vi "Multirecord Acquisition (FPGA) - custom trigger.vi"() -> ()   [LabVIEW 2021]
doc: "Use this VI as a template for the reconfigurable oscilloscope acquisition design. The block diagram is divided into three main loops.\n\nRegister Bus: This loop initializes the registers that are needed to support the configuration of the device. The FIFO bus, on the left, allows all the other design libraries to communicate with one another. This loop is very important to support the proper behavior of the instrument design library components.\n\nAcquisition: Acquires data from the I/O channels and writes the data into the record memory using the <B>Write</B> VI of the Multirecord Acquisition instrument design library. This VI also evaluates the various acquisition triggers and decides whether to acquire each data value in record memory. The host level VI (Fetch Record.vi) can read acquired records from the DRAM. The data is stored in 2 DRAM banks, each with 768 MB of storage.\n\nFetch: The recorded data is retrieved when the <B>Fetch Single Record</B> VI is run from the host VI. The <B>Write to Fetch DMA FIFO</B> VI writes data to the acq.fetch fifo 0 to transmit record data form the FPGA to the record fetch VIs on the host. This DMA FIFO must have a predefined name based on the instance parameter. By default, it is 0 (since the associated terminal on the <B>Create Resources DRAM Write Read</B> VI is unwired), so the connected FIFO is named acq.fetch fifo 0."
uses:
  Trigger/SubVIs/Types/Trigger Type.ctl
  <instrlib>/_niInstr/Data Trigger/v1/Shared/Public/Level Configuration FXP(+-,18,1).ctl
  <instrlib>/_niInstr/Data Trigger/v1/Shared/Public/Level Configuration Trigger When.ctl
  <instrlib>/_niInstr/Data Trigger/v1/Shared/Public/Edge Configuration FXP(+-,18,1).ctl
  <instrlib>/_niInstr/Data Trigger/v1/Shared/Public/Edge Configuration Trigger Slope.ctl
  FPGA Interface Typedefinitions/Trigger Combination Type.ctl
  Custom Trigger Settings.ctl
  <vilib>/Platform/TimedLoop/XDataNode/timing_clust.ctl
  <vilib>/Platform/TimedLoop/XDataNode/nitl_modes.ctl
  <vilib>/Platform/TimedLoop/XDataNode/wakeup.ctl
  <instrlib>/_niInstr/FIFO Register Bus/v1/FPGA/niInstr FIFO Register Bus v1 FPGA.lvclass
  C:/Program Files (x86)/National Instruments/LabVIEW 2021/instr.lib/_niInstr/Instruction Framework/v1/FPGA/Interfaces/Instruction Producer/Instruction Producer.lvclass
  <vilib>/rvi/Emulation/niFpgaSctlEmulationGetInTimedLoop.vi
  <vilib>/rvi/Emulation/niFpgaEmulationReportErrorSimple.vi
  <vilib>/rvi/Emulation/niFpgaGetClockAttributes.vi
  <vilib>/rvi/Emulation/niFpgaCriticalErrorInLSC.vi
  <vilib>/rvi/eio/common/nirviEmuTemplateMethod_errors.vi
  <instrlib>/HSAI-RIO/Config/Group A/v1/FPGA/Digital Correction/Validate 8 Channel Data.vi
  <instrlib>/HSAI-RIO/Config/Group A/v1/FPGA/Digital Correction/Digital Correction (8 Ch).vi
  <instrlib>/HSAI-RIO/Config/Group A/v1/FPGA/Digital Correction/FIR Filter (8 Ch).vi
  DSP/SubVIs/Integer decimationx8ch.vi
  Data Type Conversion/SubVIs/Remove Overflow FXP(+-,18,1)x8ch.vi
  Data Type Conversion/SubVIs/Data Type Conversion FXP(+-,18,1) to I16x8ch.vi
  <vilib>/Platform/TimedLoop/XDataNode/XDataNode.xnode
  <instrlib>/_niInstr/Instruction Framework/v1/FPGA/Interfaces/Address Space Collection/Address Space Collection.lvclass
  <instrlib>/_niInstr/Multirecord Acquisition/Common/v1/FPGA/niInstr Multirecord Acquisition Common v1 FPGA.lvclass
  <vilib>/eio/EIONode/EIONode.xnode
  <instrlib>/_niInstr/Instruction Framework/v1/FPGA/Top Level Bus/Register Configuration/Register Configuration.lvclass
  <vilib>/Platform/TimedLoop/XDataNode/XDNodeRunTimeDep.lvlib
  <vilib>/rvi/LocalResourceManager/LocalResourceManager.xnode
  <vilib>/rvi/eio/common/nirviEmuReportErrorAndStop.vi
  <vilib>/rvi/DataTransferAndStorage/Container/Common/niFpgaContainerGetUniqueNameForEmu.vi
  <vilib>/rvi/DataTransferAndStorage/Container/Common/niFpgaContainerSetEmuInfo.vi
  <instrlib>/_niInstr/Basic Elements/v1/FPGA/niInstr Basic Elements v1 FPGA.lvlib
  <instrlib>/_niInstr/Multirecord Acquisition/Common/v1/FPGA/Private/Create Fetch DMA FIFO Resources U8x32.vi
  <instrlib>/HSAI-RIO/Config/Group A/v1/FPGA/Digital Correction/Digital Correction.lvclass
  <instrlib>/HSAI-RIO/Config/Group A/v1/FPGA/Config Registers/Config Registers.lvclass
  <instrlib>/_niInstr/Multirecord Acquisition/Common/v1/FPGA/Private/Create Resources BRAM U384.vi
  <instrlib>/_niInstr/Multirecord Acquisition/Common/v1/FPGA/Private/Create Resources DRAM U384.vi
  <instrlib>/_niInstr/Multirecord Acquisition/Common/v1/FPGA/Private/Create Resources BRAM U768.vi
  Emulation/SubVIs/2 Element Generate Sine Cos Data FXP(+,-,14,1).vi
  C:/Program Files (x86)/National Instruments/LabVIEW 2021/instr.lib/_niInstr/FIFO Register Bus/v1/FPGA/niInstr FIFO Register Bus v1 FPGA.lvclass
  <instrlib>/_niInstr/Data Trigger/v1/Shared/niInstr Data Trigger v1 Shared.lvlib
  FPGA Interface Typedefinitions/FPGA Interface Typedefinitions.lvlib
panel:
  in  "Trigger Settings 7":T1
  in  "Trigger Settings 6":T1
  in  "Trigger Settings 5":T1
  in  "Trigger Settings 4":T1
  in  "Trigger Settings 3":T1
  in  "Trigger Settings 2":T1
  in  "Trigger Settings 1":T1
  in  "Trigger Settings 0":T1
  in  "trigger.rearm delay":u16=2
  in  "start trigger":bool=TRUE
  in  "trigger.type B":T2
  in  "reset":bool
  in  "trigger.combination type":T3
  in  "trigger.edge B":T4
  in  "trigger.level B":T6
  in  "trigger.edge A":T4
  in  "trigger.level A":T6
  in  "trigger.type A":T2
  in  "trigger.channel A":u8
  in  "trigger.channel B":u8
  out "fifo reg bus data 0":u64
  out "fifo reg bus status 0":u32
  in  "fifo reg bus ctrl 0":u32
  out "overflow":bool
  in  "dsp.decimation factor":u16
  out "overload":bool
  in  "channel.enable mask":u16=65535 format="%.0b"
  in  "channel.number of channels":u8=8
  # "Register Bus Controls"
  # "FPGA"
  # "Acquisition Loop Controls"
  # "DSP"
  # "Trigger"
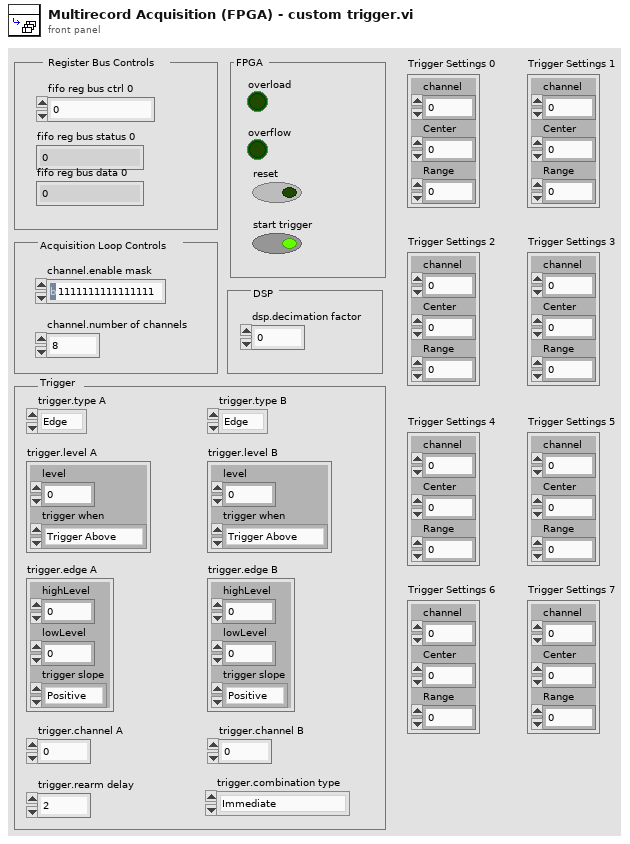
[diagram p1: front panel]
types:
  T1 = typedef "Custom Trigger Settings.ctl" = cluster{"channel":u8, "Center":fxp<+/-,24,1>, "Range":fxp<+,24,1>}
  T2 = typedef "Trigger Type.ctl" = enum16{"Edge", "Level", "Custom"}
  T3 = typedef "FPGA Interface Typedefinitions.lvlib/Trigger Combination Type.ctl" = enum16{"Immediate", "A", "B", "OR", "AND", "A THEN B", "B THEN A", "High Resolution"}
  T4 = typedef "niInstr Data Trigger v1 Shared.lvlib/Edge Configuration FXP(+-,18,1).ctl" = cluster{"highLevel":fxp<+/-,18,1>, "lowLevel":fxp<+/-,18,1>, "trigger slope":T5}
  T5 = typedef "niInstr Data Trigger v1 Shared.lvlib/Edge Configuration Trigger Slope.ctl" = enum8{"Positive", "Negative"}
  T6 = typedef "niInstr Data Trigger v1 Shared.lvlib/Level Configuration FXP(+-,18,1).ctl" = cluster{"level":fxp<+/-,18,1>, "trigger when":T7}
  T7 = typedef "niInstr Data Trigger v1 Shared.lvlib/Level Configuration Trigger When.ctl" = enum8{"Trigger Above", "Trigger Below"}
  T8 = cluster{"memory 1":refnum<k21>, "memory 2":refnum<k21>}
  T9 = typedef "XDNodeRunTimeDep.lvlib/timing_clust.ctl" = cluster{"Expected End [f-1]":u64, "Actual End [f-1]":u64, "Finished Late? [f-1]":bool, "Expected End [i-1]":u64, "Actual End [i-1]":u64, "Finished Late? [i-1]":bool, "Expected Start [i]":u64, "Actual Start [i]":u64, "Expected Start [f]":u64, "Actual Start [f]":u64, "Source Name":string, "Structure Name":string, "Period":i64, "Deadline":i64, "Offset":i64, "Start":i64, "Priority":i32, "Timeout":i32, "Mode":T10, "Wakeup Reason":T11, "Error":errorcluster, "Source Type":string, "Secondary Source Type":string, "Global End Time":u64, "Global Start Time":u64, "Frame Duration":u64, "Iteration Duration":u64, "Assigned CPU":i32, "I/O Scan Engine Mode":u32}
  T10 = typedef "XDNodeRunTimeDep.lvlib/nitl_modes.ctl" = enum32{"No Change", "Process missed periods, maintain original phase", "Discard missed periods, maintain original phase", "Process missed periods, ignore original phase", "Discard missed periods, ignore original phase"}
  T11 = typedef "XDNodeRunTimeDep.lvlib/wakeup.ctl" = enum32{"Normal", "Aborted", "Asynchronous wakeup", "Timing source error", "Timed loop error", "Timeout"}
  T12 = cluster{"Channel 0":fxp<+/-,14,1>[], "Channel 1":fxp<+/-,14,1>[], "Channel 2":fxp<+/-,14,1>[], "Channel 3":fxp<+/-,14,1>[], "Channel 4":fxp<+/-,14,1>[], "Channel 5":fxp<+/-,14,1>[], "Channel 6":fxp<+/-,14,1>[], "Channel 7":fxp<+/-,14,1>[]}
  T13 = cluster{"Channel 0":fxp<+/-,18,1>[], "Channel 1":fxp<+/-,18,1>[], "Channel 2":fxp<+/-,18,1>[], "Channel 3":fxp<+/-,18,1>[], "Channel 4":fxp<+/-,18,1>[], "Channel 5":fxp<+/-,18,1>[], "Channel 6":fxp<+/-,18,1>[], "Channel 7":fxp<+/-,18,1>[]}
  T14 = cluster{"channel 0":fxp<+/-,18,1>[], "channel 1":fxp<+/-,18,1>[], "channel 2":fxp<+/-,18,1>[], "channel 3":fxp<+/-,18,1>[], "channel 4":fxp<+/-,18,1>[], "channel 5":fxp<+/-,18,1>[], "channel 6":fxp<+/-,18,1>[], "channel 7":fxp<+/-,18,1>[]}
  T15 = cluster{"channel 0":i16[], "channel 1":i16[], "channel 2":i16[], "channel 3":i16[], "channel 4":i16[], "channel 5":i16[], "channel 6":i16[], "channel 7":i16[]}
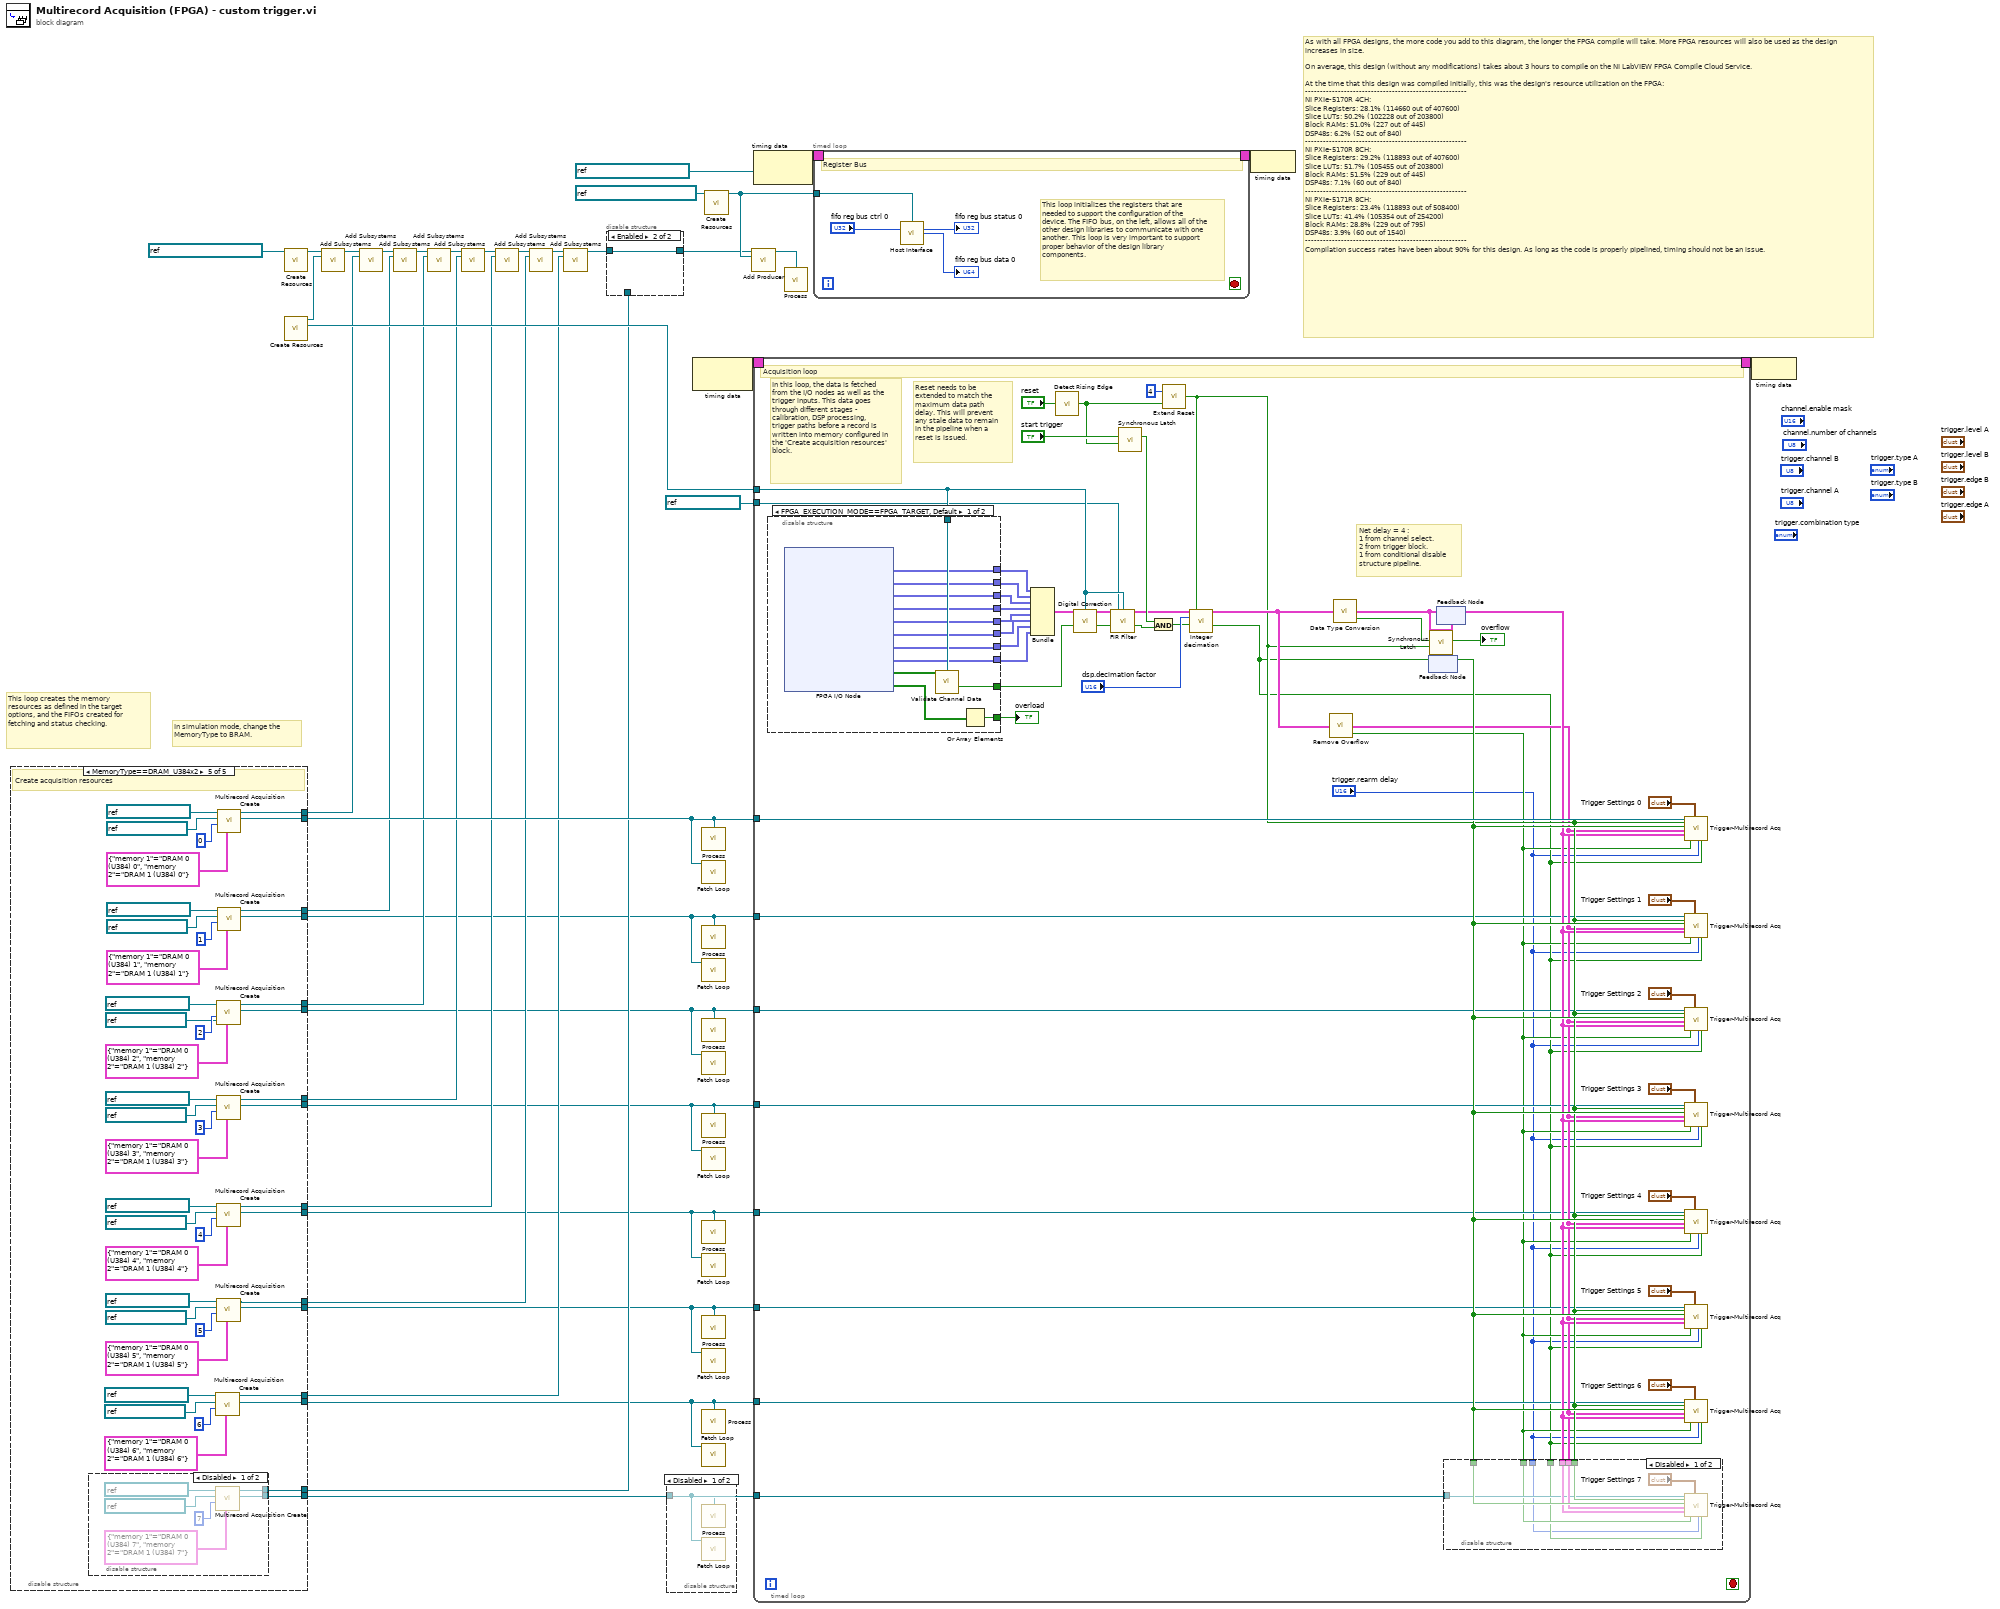
[diagram p0: block diagram]
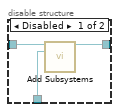
[diagram p2: hidden frame]
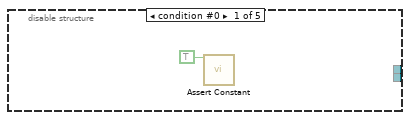
[diagram p4: hidden frame]
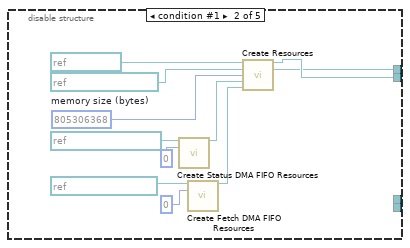
[diagram p5: hidden frame]
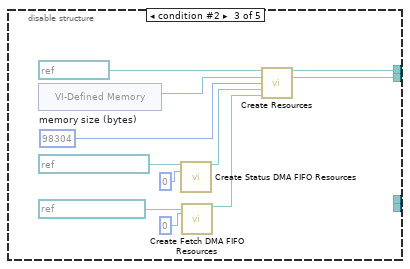
[diagram p6: hidden frame]
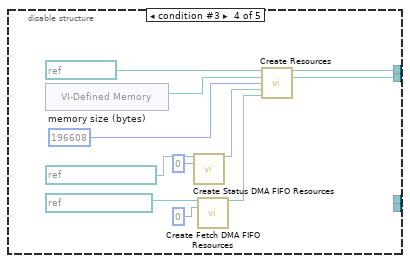
[diagram p7: hidden frame]
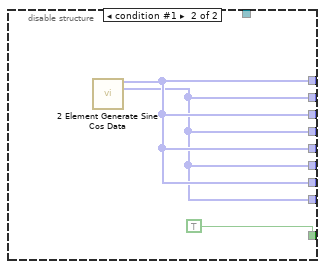
[diagram p10: hidden frame]
diagram:
  # "In simulation mode, change the MemoryType to BRAM."
  # "This loop creates the memory resources as defined in the target options, and the FIFOs created for fetching and status checking."
  # "As with all FPGA designs, the more code you add to this diagram, the longer the FPGA compile will take. More FPGA resources will also be used as the design increases in size.\n\nOn average, this design (without any modifications) takes about 3 hours to compile on the NI LabVIEW FPGA Compile Cloud Service. \n\nAt the time that this design was compiled initially, this was the design's resource utilization on the FPGA:\n------------------------------------------------------\nNI PXIe-5170R 4CH:\nSlice Registers: 28.1% (114660 out of 407600)\nSlice LUTs: 50.2% (102228 out of 203800)\nBlock RAMs: 51.0% (227 out of 445)\nDSP48s: 6.2% (52 out of 840)\n------------------------------------------------------\nNI PXIe-5170R 8CH:\nSlice Registers: 29.2% (118893 out of 407600)\nSlice LUTs: 51.7% (105455 out of 203800)\nBlock RAMs: 51.5% (229 out of 445)\nDSP48s: 7.1% (60 out of 840)\n------------------------------------------------------\nNI PXIe-5171R 8CH:\nSlice Registers: 23.4% (118893 out of 508400)\nSlice LUTs: 41.4% (105354 out of 254200)\nBlock RAMs: 28.8% (229 out of 795)\nDSP48s: 3.9% (60 out of 1540)\n------------------------------------------------------\nCompilation success rates have been about 90% for this design. As long as the code is properly pipelined, timing should not be an issue."
  n1 = disable-structure shown="MemoryType==DRAM_U384x2" {
    disable-tunnel: [_ w48 w59 w70 w116] -> w24
    disable-tunnel: [_ w45 w55 w66 w114] -> w23
    disable-tunnel: [_ _ _ _ w98] -> w22
    disable-tunnel: [_ _ _ _ w97] -> w2
    disable-tunnel: [_ _ _ _ w96] -> w16
    disable-tunnel: [_ _ _ _ w95] -> w3
    disable-tunnel: [_ _ _ _ w94] -> w14
    disable-tunnel: [_ _ _ _ w93] -> w4
    disable-tunnel: [_ _ _ _ w92] -> w13
    disable-tunnel: [_ _ _ _ w91] -> w5
    disable-tunnel: [_ _ _ _ w90] -> w12
    disable-tunnel: [_ _ _ _ w89] -> w6
    disable-tunnel: [_ _ _ _ w88] -> w11
    disable-tunnel: [_ _ _ _ w87] -> w7
    disable-tunnel: [_ _ _ _ w86] -> w9
    disable-tunnel: [_ _ _ _ w85] -> w8
    frame condition #0 {
      n2 = call <instrlib>:"Assert Constant.vi"("constant terminal"=TRUE) -> ()  [unwired: 15 in]
    }
    frame condition #1 {
      w49 = u64 805306368  # memory size (bytes)
      n3 = call <instrlib>:"Create Status DMA FIFO Resources.vi"("status dma fifo in"=refnum<k21> "acq.status fifo 0" ("status dma fifo"), "fifo instance"=u8 0) -> ("status dma fifo out"=w40:refnum<class "niInstr Status FIFO v1 FPGA.lvclass">)  [unwired: 13 in]
      n4 = call-poly <instrlib>:"Create Fetch DMA FIFO Resources.vi"("fetch dma fifo in"=refnum<k21> "acq.fetch fifo 0", "fifo instance"=u8 0) -> ("fetch dma fifo out"=w46:refnum<class "niInstr Fetch FIFO v1 FPGA.lvclass">)  [unwired: 13 in]
      n5 = call-poly <instrlib>:"Create Resources.vi"("memory clock"=refnum<k21> "160MHz" ("process clock"), "memory"=refnum<k21> "DRAM 0 (U384)" ("dram"), "memory size (bytes)"=w49, "status dma fifo resources"=w40, "fetch dma fifo resources"=w46) -> ("acquisition resources"=w48:refnum<class "niInstr Multirecord Acquisition Common v1 FPGA.lvclass">, "acquisition subsystem"=w45:refnum<class "Address Space Collection.lvclass">)  [unwired: 9 in]
    }
    frame condition #2 {
      w60 = u64 98304  # memory size (bytes)
      n6 = xnode "VI-Defined Memory"() -> ("Memory Out"=w61:refnum<k21>)
      n7 = call <instrlib>:"Create Status DMA FIFO Resources.vi"("status dma fifo in"=refnum<k21> "acq.status fifo 0" ("status dma fifo"), "fifo instance"=u8 0) -> ("status dma fifo out"=w52:refnum<class "niInstr Status FIFO v1 FPGA.lvclass">)  [unwired: 13 in]
      n8 = call-poly <instrlib>:"Create Fetch DMA FIFO Resources.vi"("fetch dma fifo in"=refnum<k21> "acq.fetch fifo 0", "fifo instance"=u8 0) -> ("fetch dma fifo out"=w56:refnum<class "niInstr Fetch FIFO v1 FPGA.lvclass">)  [unwired: 13 in]
      n9 = call-poly <instrlib>:"Create Resources.vi"("memory clock"=refnum<k21> "160MHz" ("process clock"), "memory"=w61, "memory size (bytes)"=w60, "status dma fifo resources"=w52, "fetch dma fifo resources"=w56) -> ("acquisition resources"=w59:refnum<class "niInstr Multirecord Acquisition Common v1 FPGA.lvclass">, "acquisition subsystem"=w55:refnum<class "Address Space Collection.lvclass">)  [unwired: 9 in]
    }
    frame condition #3 {
      w71 = u64 196608  # memory size (bytes)
      n10 = xnode "VI-Defined Memory"() -> ("Memory Out"=w72:refnum<k21>)
      n11 = call <instrlib>:"Create Status DMA FIFO Resources.vi"("status dma fifo in"=refnum<k21> "acq.status fifo 0" ("status dma fifo"), "fifo instance"=u8 0) -> ("status dma fifo out"=w64:refnum<class "niInstr Status FIFO v1 FPGA.lvclass">)  [unwired: 13 in]
      n12 = call-poly <instrlib>:"Create Fetch DMA FIFO Resources.vi"("fetch dma fifo in"=refnum<k21> "acq.fetch fifo 0", "fifo instance"=u8 0) -> ("fetch dma fifo out"=w67:refnum<class "niInstr Fetch FIFO v1 FPGA.lvclass">)  [unwired: 13 in]
      n13 = call-poly <instrlib>:"Create Resources.vi"("memory clock"=refnum<k21> "160MHz" ("process clock"), "memory"=w72, "memory size (bytes)"=w71, "status dma fifo resources"=w64, "fetch dma fifo resources"=w67) -> ("acquisition resources"=w70:refnum<class "niInstr Multirecord Acquisition Common v1 FPGA.lvclass">, "acquisition subsystem"=w66:refnum<class "Address Space Collection.lvclass">)  [unwired: 9 in]
    }
    frame condition #4 (active) {
      # "Create acquisition resources"
      n14 = disable-structure shown="Disabled" {
        disable-tunnel: [w122 _] -> w86
        disable-tunnel: [w121 _] -> w85
        frame Disabled {
          n15 = call "Multirecord Acquisition Create.vi"("DRAM"=T8 {"memory 1"="DRAM 0 (U384) 7", "memory 2"="DRAM 1 (U384) 7"} ("memory"), "instance"=u8 7, "acq.fetch fifo in"=refnum<k21> "acq.fetch fifo 7" ("fetch dma fifo in"), "acq.status fifo in"=refnum<k21> "acq.status fifo 7" ("status dma fifo")) -> ("acquisition resources"=w121:refnum<class "niInstr Multirecord Acquisition Common v1 FPGA.lvclass">, "Address Space Collection out"=w122:refnum<class "Address Space Collection.lvclass">)  [unwired: 6 in]
        }
        frame Enabled {
        }
      }
      n16 = call "Multirecord Acquisition Create.vi"("DRAM"=T8 {"memory 1"="DRAM 0 (U384) 6", "memory 2"="DRAM 1 (U384) 6"} ("memory"), "instance"=u8 6, "acq.fetch fifo in"=refnum<k21> "acq.fetch fifo 6" ("fetch dma fifo in"), "acq.status fifo in"=refnum<k21> "acq.status fifo 6" ("status dma fifo")) -> ("acquisition resources"=w87:refnum<class "niInstr Multirecord Acquisition Common v1 FPGA.lvclass">, "Address Space Collection out"=w88:refnum<class "Address Space Collection.lvclass">)  [unwired: 6 in]
      n17 = call "Multirecord Acquisition Create.vi"("DRAM"=T8 {"memory 1"="DRAM 0 (U384) 2", "memory 2"="DRAM 1 (U384) 2"} ("memory"), "instance"=u8 2, "acq.fetch fifo in"=refnum<k21> "acq.fetch fifo 2" ("fetch dma fifo in"), "acq.status fifo in"=refnum<k21> "acq.status fifo 2" ("status dma fifo")) -> ("acquisition resources"=w95:refnum<class "niInstr Multirecord Acquisition Common v1 FPGA.lvclass">, "Address Space Collection out"=w96:refnum<class "Address Space Collection.lvclass">)  [unwired: 6 in]
      n18 = call "Multirecord Acquisition Create.vi"("DRAM"=T8 {"memory 1"="DRAM 0 (U384) 3", "memory 2"="DRAM 1 (U384) 3"} ("memory"), "instance"=u8 3, "acq.fetch fifo in"=refnum<k21> "acq.fetch fifo 3" ("fetch dma fifo in"), "acq.status fifo in"=refnum<k21> "acq.status fifo 3" ("status dma fifo")) -> ("acquisition resources"=w93:refnum<class "niInstr Multirecord Acquisition Common v1 FPGA.lvclass">, "Address Space Collection out"=w94:refnum<class "Address Space Collection.lvclass">)  [unwired: 6 in]
      n19 = call "Multirecord Acquisition Create.vi"("DRAM"=T8 {"memory 1"="DRAM 0 (U384) 4", "memory 2"="DRAM 1 (U384) 4"} ("memory"), "instance"=u8 4, "acq.fetch fifo in"=refnum<k21> "acq.fetch fifo 4" ("fetch dma fifo in"), "acq.status fifo in"=refnum<k21> "acq.status fifo 4" ("status dma fifo")) -> ("acquisition resources"=w91:refnum<class "niInstr Multirecord Acquisition Common v1 FPGA.lvclass">, "Address Space Collection out"=w92:refnum<class "Address Space Collection.lvclass">)  [unwired: 6 in]
      n20 = call "Multirecord Acquisition Create.vi"("DRAM"=T8 {"memory 1"="DRAM 0 (U384) 5", "memory 2"="DRAM 1 (U384) 5"} ("memory"), "instance"=u8 5, "acq.fetch fifo in"=refnum<k21> "acq.fetch fifo 5" ("fetch dma fifo in"), "acq.status fifo in"=refnum<k21> "acq.status fifo 5" ("status dma fifo")) -> ("acquisition resources"=w89:refnum<class "niInstr Multirecord Acquisition Common v1 FPGA.lvclass">, "Address Space Collection out"=w90:refnum<class "Address Space Collection.lvclass">)  [unwired: 6 in]
      n21 = call "Multirecord Acquisition Create.vi"("DRAM"=T8 {"memory 1"="DRAM 0 (U384) 0", "memory 2"="DRAM 1 (U384) 0"} ("memory"), "instance"=u8 0, "acq.fetch fifo in"=refnum<k21> "acq.fetch fifo 0" ("fetch dma fifo in"), "acq.status fifo in"=refnum<k21> "acq.status fifo 0" ("status dma fifo")) -> ("acquisition resources"=w116:refnum<class "niInstr Multirecord Acquisition Common v1 FPGA.lvclass">, "Address Space Collection out"=w114:refnum<class "Address Space Collection.lvclass">)  [unwired: 6 in]
      n22 = call "Multirecord Acquisition Create.vi"("DRAM"=T8 {"memory 1"="DRAM 0 (U384) 1", "memory 2"="DRAM 1 (U384) 1"} ("memory"), "instance"=u8 1, "acq.fetch fifo in"=refnum<k21> "acq.fetch fifo 1" ("fetch dma fifo in"), "acq.status fifo in"=refnum<k21> "acq.status fifo 1" ("status dma fifo")) -> ("acquisition resources"=w97:refnum<class "niInstr Multirecord Acquisition Common v1 FPGA.lvclass">, "Address Space Collection out"=w98:refnum<class "Address Space Collection.lvclass">)  [unwired: 6 in]
    }
  }
  n23 = call <instrlib>:"Create Resources.vi"("register clock"=refnum<k21> "40 MHz Onboard Clock" ("Source Name")) -> ("register configuration"=w31:refnum<class "Register Configuration.lvclass">)  [unwired: 14 in]
  n24 = call <instrlib>:"Create Resources.vi"() -> ("config subsystems"=w29:refnum<class "Address Space Collection.lvclass">, "digital correction resources"=w25:refnum<class "Digital Correction.lvclass">)  [unwired: 14 in]
  n25 = call-dynamic "Add Subsystems.vi"("register configuration in"=w31, "subsystems"=w29) -> ("register configuration out"=w30:refnum<class "Register Configuration.lvclass">)  [unwired: 13 in]
  n26 = call-dynamic "Add Subsystems.vi"("register configuration in"=w30, "subsystems"=w23) -> ("register configuration out"=w21:refnum<class "Register Configuration.lvclass">)  [unwired: 13 in]
  n27 = call-dynamic "Add Subsystems.vi"("register configuration in"=w21, "subsystems"=w22) -> ("register configuration out"=w15:refnum<class "Register Configuration.lvclass">)  [unwired: 13 in]
  n28 = call-dynamic "Add Subsystems.vi"("register configuration in"=w15, "subsystems"=w16) -> ("register configuration out"=w20:refnum<class "Register Configuration.lvclass">)  [unwired: 13 in]
  n29 = call-dynamic "Add Subsystems.vi"("register configuration in"=w20, "subsystems"=w14) -> ("register configuration out"=w18:refnum<class "Register Configuration.lvclass">)  [unwired: 13 in]
  n30 = call-dynamic "Add Subsystems.vi"("register configuration in"=w18, "subsystems"=w13) -> ("register configuration out"=w19:refnum<class "Register Configuration.lvclass">)  [unwired: 13 in]
  n31 = call-dynamic "Add Subsystems.vi"("register configuration in"=w19, "subsystems"=w12) -> ("register configuration out"=w10:refnum<class "Register Configuration.lvclass">)  [unwired: 13 in]
  n32 = call-dynamic "Add Subsystems.vi"("register configuration in"=w10, "subsystems"=w11) -> ("register configuration out"=w1:refnum<class "Register Configuration.lvclass">)  [unwired: 13 in]
  n33 = disable-structure shown="Enabled" {
    disable-tunnel: [w125 w126] -> w17
    disable-tunnel: w9 -> [w124 _]
    disable-tunnel: w1 -> [w123 w126]
    frame Disabled {
      n34 = call-dynamic "Add Subsystems.vi"("register configuration in"=w123, "subsystems"=w124) -> ("register configuration out"=w125:refnum<class "Register Configuration.lvclass">)  [unwired: 13 in]
    }
    frame Enabled {
    }
  }
  n35 = disable-structure shown="Disabled" {
    disable-tunnel: w8 -> [w127 _]
    frame Disabled {
      n36 = call-dynamic "Process.vi"("acquisition resources"=w127) -> ()  [unwired: 15 in]
      n37 = call "Fetch Loop.vi"("niInstr Multirecord Acquisition Common v1 FPGA in"=w127) -> ()  [unwired: 11 in]
    }
    frame Enabled {
    }
  }
  n38 = node-c288() -> (w36:T9)  [unwired: 1 in]
  n39 = call-dynamic "Process.vi"("acquisition resources"=w24) -> ()  [unwired: 15 in]
  n40 = call "Fetch Loop.vi"("niInstr Multirecord Acquisition Common v1 FPGA in"=w24) -> ()  [unwired: 11 in]
  n41 = call-dynamic "Process.vi"("acquisition resources"=w2) -> ()  [unwired: 15 in]
  n42 = call "Fetch Loop.vi"("niInstr Multirecord Acquisition Common v1 FPGA in"=w2) -> ()  [unwired: 11 in]
  n43 = call-dynamic "Process.vi"("acquisition resources"=w3) -> ()  [unwired: 15 in]
  n44 = call "Fetch Loop.vi"("niInstr Multirecord Acquisition Common v1 FPGA in"=w3) -> ()  [unwired: 11 in]
  n45 = call-dynamic "Process.vi"("acquisition resources"=w4) -> ()  [unwired: 15 in]
  n46 = call "Fetch Loop.vi"("niInstr Multirecord Acquisition Common v1 FPGA in"=w4) -> ()  [unwired: 11 in]
  n47 = call-dynamic "Process.vi"("acquisition resources"=w5) -> ()  [unwired: 15 in]
  n48 = call "Fetch Loop.vi"("niInstr Multirecord Acquisition Common v1 FPGA in"=w5) -> ()  [unwired: 11 in]
  n49 = call-dynamic "Process.vi"("acquisition resources"=w6) -> ()  [unwired: 15 in]
  n50 = call "Fetch Loop.vi"("niInstr Multirecord Acquisition Common v1 FPGA in"=w6) -> ()  [unwired: 11 in]
  n51 = call-dynamic "Process.vi"("acquisition resources"=w7) -> ()  [unwired: 15 in]
  n52 = call "Fetch Loop.vi"("niInstr Multirecord Acquisition Common v1 FPGA in"=w7) -> ()  [unwired: 11 in]
  n53 = call <instrlib>:"Create Resources.vi"("instruction fifo"=refnum<k21> "reg.host instruction fifo 0" ("FIFO")) -> ("fifo register bus"=w28:refnum<class "niInstr FIFO Register Bus v1 FPGA.lvclass">)  [unwired: 14 in]
  n54 = call-dynamic "Add Producer.vi"("register configuration in"=w17, "instruction producer"=w28) -> ("register configuration out"=w27:refnum<class "Register Configuration.lvclass">)  [unwired: 13 in]
  n55 = node-c288(refnum<k21> "40 MHz Onboard Clock" ("Source Name")) -> (w38:T9)
  n56 = timed-loop {
    timing: w36 -> [_]
    timing-out: [_] -> w35
    tunnel: w24 -> [w177]
    tunnel: w25 -> [w170]
    tunnel: refnum<k21> "Data Clock x2" -> [w167]
    tunnel: w8 -> [w140]
    tunnel: w7 -> [w139]
    tunnel: w6 -> [w138]
    tunnel: w5 -> [w137]
    tunnel: w4 -> [w136]
    tunnel: w3 -> [w135]
    tunnel: w2 -> [w134]
    stop <- _ stop-if-true
    # "Net delay = 4 :\n1 from channel select.\n2 from trigger block.\n1 from conditional disable structure pipeline."
    # "Reset needs to be extended to match the maximum data path delay. This will prevent any stale data to remain in the pipeline when a reset is issued."
    # "In this loop, the data is fetched from the I/O nodes as well as the trigger inputs. This data goes through different stages - calibration, DSP processing, trigger paths before a record is written into memory configured in the 'Create acquisition resources' block."
    # "Acquisition loop"
    n57 = disable-structure shown="FPGA_EXECUTION_MODE==FPGA_TARGET, Default" {
      disable-tunnel: [w197 w202] -> w166
      disable-tunnel: [w196 w201] -> w165
      disable-tunnel: [w195 w202] -> w164
      disable-tunnel: [w194 w201] -> w163
      disable-tunnel: [w193 w202] -> w162
      disable-tunnel: [w192 w201] -> w161
      disable-tunnel: [w191 w202] -> w159
      disable-tunnel: [w190 w201] -> w160
      disable-tunnel: [w187 TRUE ("ADC Data Valid")] -> w157
      disable-tunnel: w170 -> [w198 _]
      disable-tunnel: [w188 _] -> w176
      frame condition #0 (active) {
        # "I/O Nodes"
        n58 = xnode "FPGA I/O Node"() -> ("Channel 0"=w197:fxp<+/-,14,1>[], "Channel 1"=w196:fxp<+/-,14,1>[], "Channel 2"=w195:fxp<+/-,14,1>[], "Channel 3"=w194:fxp<+/-,14,1>[], "Channel 4"=w193:fxp<+/-,14,1>[], "Channel 5"=w192:fxp<+/-,14,1>[], "Channel 6"=w191:fxp<+/-,14,1>[], "Channel 7"=w190:fxp<+/-,14,1>[], "Channel Data Valid"=w199:bool[], "Channel Overload"=w189:bool[])  [unwired: 10 in, 10 out]
        n59 = call-poly <instrlib>:"Validate Channel Data.vi"("channel data valid"=w199, "digital correction resources"=w198) -> ("expected data valid"=w187:bool)  [unwired: 13 in]
        n60 = Or Array Elements(Boolean array=w189) -> (logical OR=w188:bool)
      }
      frame condition #1 {
        n61 = call-poly "2 Element Generate Sine Cos Data.vi"() -> ("sine data"=w202:fxp<+/-,14,1>[], "cosine data"=w201:fxp<+/-,14,1>[])  [unwired: 14 in]
      }
    }
    "overload" <- w176
    n62 = Bundle("Channel 0"=w166, "Channel 1"=w165, "Channel 2"=w164, "Channel 3"=w163, "Channel 4"=w162, "Channel 5"=w161, "Channel 6"=w159, "Channel 7"=w160) -> (w158:T12)  [unwired: 1 in]
    n63 = call <instrlib>:"Detect Rising Edge.vi"("signal"="reset") -> ("edge detected"=w169:bool)  [unwired: 14 in]
    n64 = call-poly <instrlib>:"Digital Correction.vi"("channel data in"=w158, "digital correction resources"=w170, "input valid"=w157) -> ("corrected channel data out"=w152:T13, "output valid"=w151:bool)  [unwired: 11 in]
    n65 = call-poly <instrlib>:"FIR Filter.vi"("data in"=w152, "data clock x2"=w167, "digital correction resources"=w170, "input valid"=w151) -> ("data out"=w149:T13, "output valid"=w150:bool)  [unwired: 9 in, 1 out]
    n66 = call <instrlib>:"Synchronous Latch.vi"("clear"=w169, "set"="start trigger") -> ("out"=w172:bool)  [unwired: 9 in]
    n67 = And(x=w172, y=w150) -> (x .and. y?=w153:bool)
    n68 = call "Extend Reset.vi"("reset in"=w169, "number of cycles"=u8 4) -> ("reset out"=w143:bool)
    n69 = call-poly "Integer decimation.vi"("data in"=w149, "reset"=w143, "decimation factor"="dsp.decimation factor", "input valid"=w153) -> ("data out"=w155:T14, "output valid"=w132:bool)  [unwired: 9 in, 1 out]
    n70 = call-poly "Remove Overflow.vi"("data in"=w155) -> ("overflow"=w133:bool, "data out"=w141:T14)  [unwired: 3 in]
    n71 = call-poly "Data Type Conversion.vi"("data in"=w155) -> ("overflow"=w156:bool, "data out"=w154:T15)  [unwired: 3 in]
    n72 = feedback #1() -> (w144:bool)  [unwired: 1 in]
    n73 = feedback-in #1(w132) -> ()
    n74 = call <instrlib>:"Synchronous Latch.vi"("clear"=w143, "set"=w156) -> ("out"=→"overflow":bool)  [unwired: 9 in]
    n75 = feedback #2(w154) -> (w142:T15)
    n76 = feedback-in #2(w154) -> ()
    n77 = disable-structure shown="Disabled" {
      disable-tunnel: w144 -> [w186 _]
      disable-tunnel: w143 -> [w185 _]
      disable-tunnel: w142 -> [w184 _]
      disable-tunnel: w141 -> [w183 _]
      disable-tunnel: w140 -> [w182 _]
      disable-tunnel: w133 -> [w181 _]
      disable-tunnel: w132 -> [w180 _]
      disable-tunnel: "trigger.rearm delay" -> [w179 _]
      frame Disabled {
        n78 = call "Trigger-Multirecord Acq.vi"("niInstr Multirecord Acquisition Common v1 FPGA in"=w182, "reset in"=w185, "Ch. correction output valid"=w186, "trigger data in"=w183, "data in"=w184, "overflow"=w181, "Trigger Settings"="Trigger Settings 7", "trigger.rearm delay"=w179, "Trigger Data  input valid"=w180) -> ()  [unwired: 7 in, 4 out]
      }
      frame Enabled {
      }
    }
    n79 = call "Trigger-Multirecord Acq.vi"("niInstr Multirecord Acquisition Common v1 FPGA in"=w177, "reset in"=w143, "Ch. correction output valid"=w144, "trigger data in"=w141, "data in"=w142, "overflow"=w133, "Trigger Settings"="Trigger Settings 0", "trigger.rearm delay"="trigger.rearm delay", "Trigger Data  input valid"=w132) -> ()  [unwired: 7 in, 4 out]
    n80 = call "Trigger-Multirecord Acq.vi"("niInstr Multirecord Acquisition Common v1 FPGA in"=w134, "reset in"=w143, "Ch. correction output valid"=w144, "trigger data in"=w141, "data in"=w142, "overflow"=w133, "Trigger Settings"="Trigger Settings 1", "trigger.rearm delay"="trigger.rearm delay", "Trigger Data  input valid"=w132) -> ()  [unwired: 7 in, 4 out]
    n81 = call "Trigger-Multirecord Acq.vi"("niInstr Multirecord Acquisition Common v1 FPGA in"=w135, "reset in"=w143, "Ch. correction output valid"=w144, "trigger data in"=w141, "data in"=w142, "overflow"=w133, "Trigger Settings"="Trigger Settings 2", "trigger.rearm delay"="trigger.rearm delay", "Trigger Data  input valid"=w132) -> ()  [unwired: 7 in, 4 out]
    n82 = call "Trigger-Multirecord Acq.vi"("niInstr Multirecord Acquisition Common v1 FPGA in"=w136, "reset in"=w143, "Ch. correction output valid"=w144, "trigger data in"=w141, "data in"=w142, "overflow"=w133, "Trigger Settings"="Trigger Settings 3", "trigger.rearm delay"="trigger.rearm delay", "Trigger Data  input valid"=w132) -> ()  [unwired: 7 in, 4 out]
    n83 = call "Trigger-Multirecord Acq.vi"("niInstr Multirecord Acquisition Common v1 FPGA in"=w137, "reset in"=w143, "Ch. correction output valid"=w144, "trigger data in"=w141, "data in"=w142, "overflow"=w133, "Trigger Settings"="Trigger Settings 4", "trigger.rearm delay"="trigger.rearm delay", "Trigger Data  input valid"=w132) -> ()  [unwired: 7 in, 4 out]
    n84 = call "Trigger-Multirecord Acq.vi"("niInstr Multirecord Acquisition Common v1 FPGA in"=w138, "reset in"=w143, "Ch. correction output valid"=w144, "trigger data in"=w141, "data in"=w142, "overflow"=w133, "Trigger Settings"="Trigger Settings 5", "trigger.rearm delay"="trigger.rearm delay", "Trigger Data  input valid"=w132) -> ()  [unwired: 7 in, 4 out]
    n85 = call "Trigger-Multirecord Acq.vi"("niInstr Multirecord Acquisition Common v1 FPGA in"=w139, "reset in"=w143, "Ch. correction output valid"=w144, "trigger data in"=w141, "data in"=w142, "overflow"=w133, "Trigger Settings"="Trigger Settings 6", "trigger.rearm delay"="trigger.rearm delay", "Trigger Data  input valid"=w132) -> ()  [unwired: 7 in, 4 out]
  }
  n86 = call-dynamic "Process.vi"("register configuration"=w27) -> ()  [unwired: 15 in]
  n87 = timed-loop {
    timing: w38 -> [_]
    timing-out: [_] -> w37
    tunnel: w28 -> [w208]
    stop <- _ stop-if-true
    # "This loop initializes the registers that are needed to support the configuration of the device. The FIFO bus, on the left, allows all of the other design libraries to communicate with one another. This loop is very important to support proper behavior of the design library components."
    # "Register Bus"
    n88 = call <instrlib>:"Host Interface.vi"("fifo register bus"=w208, "fifo reg bus ctrl 0"="fifo reg bus ctrl 0") -> ("fifo reg bus status 0"=→"fifo reg bus status 0":u32, "fifo reg bus data 0"=→"fifo reg bus data 0":u64)  [unwired: 12 in]
  }
  n89 = node-c288(w37) -> ()
  n90 = node-c288(w35) -> ()
